vi "Do.vi"(8 "error in (no error)":errorcluster, 10 "Actor in":refnum<class "Actor.lvclass">, 11 "Balance_abs Msg":refnum<class "Balance_abs Msg.lvclass">) -> (0 "error out":errorcluster, 2 "Actor out":refnum<class "Actor.lvclass">)   [LabVIEW 2025, in "UserConsole.lvlib" / "Balance_abs Msg.lvclass"]
doc: "This VI delivers the message to the actor by calling the appropriate method(s) on the actor."
uses:
  Balance_abs Msg.lvclass
  Balance_abs Msg.lvclass/Balance_abs Msg.ctl
  C:/Users/halstead_rideriver/Documents/Labview_Practice/ATM_Machine_Actor Framework/ATM_ACTOR_Without_States/Database_handler/Database_handler Messages/Amt_fb_user Msg/Amt_fb_user Msg.lvclass
  C:/Program Files (x86)/National Instruments/LabVIEW 2025/vi.lib/ActorFramework/Message/Message.lvclass
  C:/Users/halstead_rideriver/Documents/Labview_Practice/ATM_Machine_Actor Framework/ATM_ACTOR_Without_States/UserConsole Messages/Balance_abs Msg/Balance_abs Msg.lvclass
  34700b1e-4b1b-4205-ab4b-28631ba2a4c6.vi
  UserConsole/UserConsole.lvclass
  Database_handler/Database_handler Messages/Amt_fb_user Msg/Amt_fb_user Msg.lvclass
  <vilib>/ActorFramework/Actor/Actor.lvclass
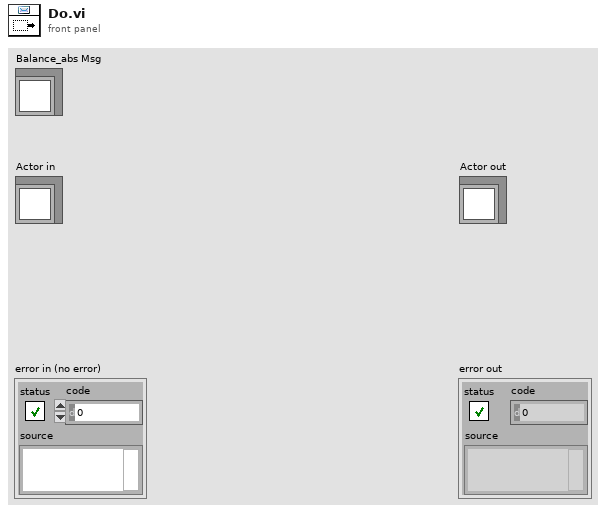
[diagram p1: front panel]
types:
  T1 = cluster{"Database":cluster{"Balance":dbl, "Password":string}}
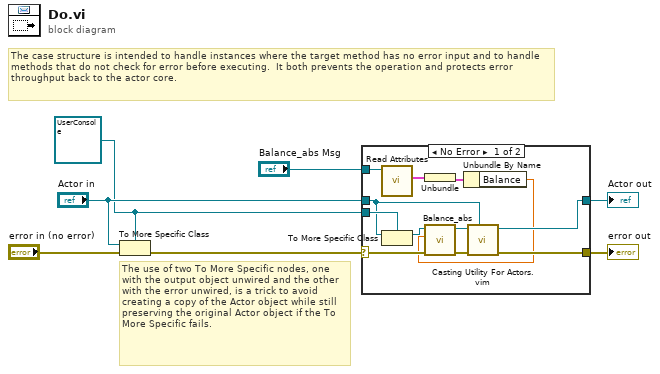
[diagram p0: block diagram]
diagram:
  w2 = refnum<class "UserConsole.lvclass"> refnum ("Actor in")
  # "The use of two To More Specific nodes, one with the output object unwired and the other with the error unwired, is a trick to avoid creating a copy of the Actor object while still preserving the original Actor object if the To More Specific fails."
  # "The case structure is intended to handle instances where the target method has no error input and to handle methods that do not check for error before executing.  It both prevents the operation and protects error throughput back to the actor core."
  n1 = To More Specific Class(target class=w2, reference="Actor in", error in="error in (no error)") -> (error out=w6:errorcluster)  [unwired: 1 out]
  n2 = case shown="No Error" w6 {
    selector: w6 -> [w19 w21]
    tunnel: [w11 w21] -> w5
    tunnel: [w10 w20] -> w4
    tunnel: "Actor in" -> [w14 w20]
    tunnel: w2 -> [w15 _]
    tunnel: "Balance_abs Msg" -> [w16 _]
    frame No Error {
      n3 = call "Read Attributes.vi"("Amt_fb_user Msg"=w16) -> ("Payload"=w17:T1)  [unwired: 10 in]
      n4 = To More Specific Class(target class=w15, reference=w14) -> (specific class reference=w18:refnum<class "UserConsole.lvclass">)  [unwired: 1 in, 1 out]
      n5 = Unbundle(w17) -> ("Database"=w9:cluster{"Balance":dbl, "Password":string})
      n6 = Unbundle By Name(w9) -> ("Balance"=w8:dbl)
      n7 = call-dynamic "Balance_abs.vi"("error in (no error)"=w19, "Balance"=w8, "UserConsole in"=w18) -> ("error out"=w12:errorcluster, "UserConsole out"=w13:refnum<class "UserConsole.lvclass">)  [unwired: 7 in]
      n8 = call "Casting Utility For Actors.vim"("type"=w14, "error in (no error)"=w12, "Actor in"=w13) -> ("error out"=w11:errorcluster, "Actor out"=w10:refnum<class "Actor.lvclass">)  [unwired: 7 in]
    }
    frame Error {
      # "If type check fails, pass the original object out again."
    }
  }
  "error out" <- w5
  "Actor out" <- w4
